vi "HTTP Error.vi"(8 "error in (no error)":errorcluster, 10 "Body":string, 11 "Header":string) -> (0 "error out":errorcluster, 2 "Success?":bool, 3 "HTTP Error Code":i32)   [LabVIEW 2011, in "i3-twitter.lvlib"]
doc: "Get HTTP error code and body, if any."
uses:
  i3-twitter.lvlib
  <vilib>/Utility/error.llb/whitespace.ctl
  i3-json/JSON Parsing/Get Object Parameter Files/Get Object Parameter - Array.vi
  i3-json/JSON Parsing/Get Array Value at Index Files/Get Array Value at Index - Object.vi
  i3-json/JSON Parsing/Get Object Parameter Files/Get Object Parameter - String.vi
  i3-json/JSON Parsing/Get Object Parameter Files/Get Object Parameter - Numeric.vi
  i3-json/i3-json.lvlib
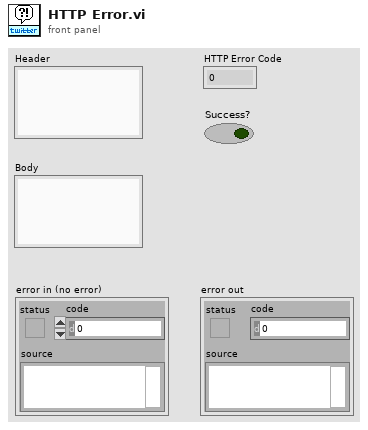
[diagram p1: front panel]
types:
  T1 = typedef "whitespace.ctl" = u16
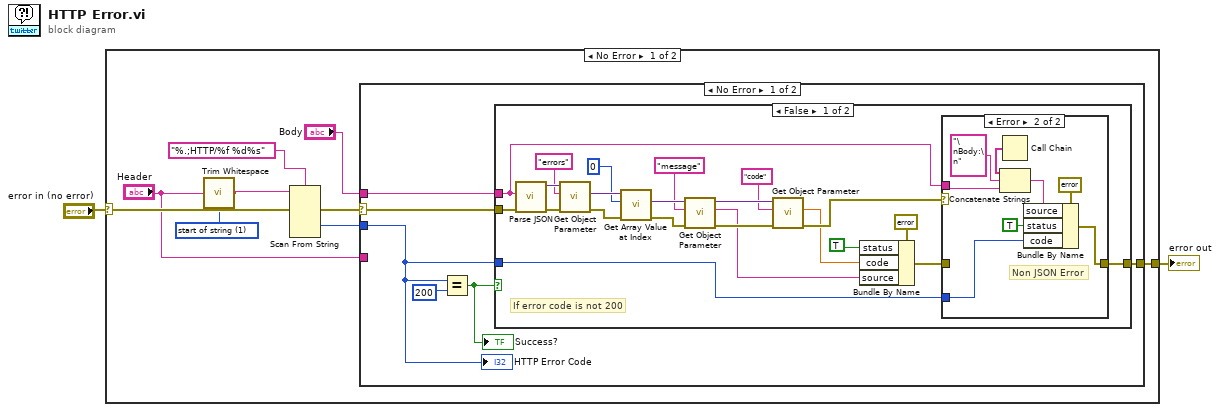
[diagram p0: block diagram]
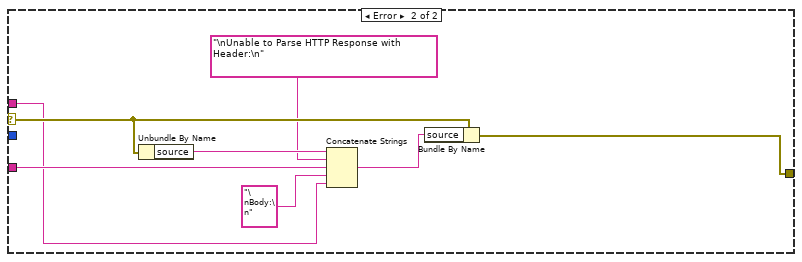
[diagram p4: hidden frame]
diagram:
  n1 = case shown="No Error" "error in (no error)" {
    selector: "error in (no error)" -> [w9 w58]
    tunnel: [w8 w58] -> w1
    frame No Error {
      w4 = T1 1 items=["both", "start of string", "end of string"] ("location (both)")
      n2 = call <vilib>:"Trim Whitespace.vi"("string"="Header", "location (both)"=w4) -> ("trimmed string"=w5:string)
      n3 = Scan From String(format string="%.;HTTP/%f %d%s", input string=w5, error in=w9) -> (error out=w7:errorcluster, output 2=w11:i32)  [unwired: 6 in, 2 out]
      n4 = case shown="No Error" w7 {
        selector: w7 -> [w13 w57]
        tunnel: w11 -> [w17 _]
        tunnel: [w14 w53] -> w8
        tunnel: "Header" -> [_ w52]
        tunnel: "Body" -> [w12 w50]
        frame No Error {
          n5 = Equal?(x=w17, y=200) -> (x = y?=w16:bool)
          "Success?" <- w16
          n6 = case shown="False" w16 {
            tunnel: [w19 w49] -> w14
            tunnel: w13 -> [w31 w49]
            tunnel: w17 -> [w18 _]
            tunnel: w12 -> [w20 _]
            frame False {
              # "If error code is not 200"
              n7 = call "Parse JSON.vi"("error in (no error)"=w31, "JSON String"=w20) -> ("error out"=w30:errorcluster, "JSON Tree"=w33:variant)  [unwired: 6 in, 2 out]
              n8 = call-poly "Get Object Parameter.vi"("error in (no error)"=w30, "Parameter Name"="errors", "JSON Tree In (JSON Object)"=w33) -> ("error out"=w29:errorcluster, "JSON Array"=w37:variant)  [unwired: 5 in, 2 out]
              n9 = call-poly "Get Array Value at Index.vi"("error in (no error)"=w29, "Index"=0, "JSON Tree In (JSON Array)"=w37) -> ("error out"=w27:errorcluster, "JSON Object"=w38:variant)  [unwired: 5 in, 2 out]
              n10 = call-poly "Get Object Parameter.vi"("error in (no error)"=w27, "Parameter Name"="message", "JSON Tree In (JSON Object)"=w38) -> ("error out"=w26:errorcluster, "String Value"=w23:string, "JSON Tree Out Passthrough"=w36:variant)  [unwired: 5 in, 1 out]
              n11 = call-poly "Get Object Parameter.vi"("error in (no error)"=w26, "Parameter Name"="code", "JSON Tree In (JSON Object)"=w36) -> ("error out"=w39:errorcluster, "Double Value"=w22:dbl)  [unwired: 5 in, 2 out]
              n12 = Bundle By Name(cluster=errorcluster {"status"=FALSE, "code"=0, "source"=""} ("error constant"), "status"=TRUE, "code"=w22, "source"=w23) -> (w21:errorcluster)
              n13 = case shown="Error" w39 {
                tunnel: w21 -> [w40 _]
                tunnel: w20 -> [_ w42]
                tunnel: [w40 w47] -> w19
                tunnel: w18 -> [_ w41]
                frame No Error {
                  # "Standard Twitter\nJSON Error"
                }
                frame Error {
                  # "Non JSON Error"
                  n14 = Call Chain() -> (call chain=w44:string[])
                  n15 = Concatenate Strings(w44, "\nBody:\n" ("string"), w42) -> (w45:string)
                  n16 = Bundle By Name(cluster=errorcluster {"status"=FALSE, "code"=0, "source"=""} ("error constant"), "source"=w45, "status"=TRUE, "code"=w41) -> (w47:errorcluster)
                }
              }
            }
            frame True {
              # "Success is True"
            }
          }
          "HTTP Error Code" <- w17
        }
        frame Error {
          n17 = Unbundle By Name(w57) -> ("source"=w56:string)
          n18 = Concatenate Strings(w56, "\nUnable to Parse HTTP Response with Header:\n" ("string"), w52, "\nBody:\n" ("string"), w50) -> (w54:string)
          n19 = Bundle By Name(cluster=w57, "source"=w54) -> (w53:errorcluster)
        }
      }
    }
    frame Error {
    }
  }
  "error out" <- w1
